vi "Begin Map.vi"   [LabVIEW 2017, in "LabPack.lvlib" / "Writer.lvclass"]
doc: "Starts writing and encoding a series of key-value pairs (ma) to MessagePack binary data format."
uses:
  Writer.lvclass
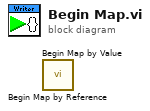
[diagram p0: block diagram]
diagram:
  n1 = call "Begin Map by Reference.vi"() -> ()  [unwired: 10 in, 2 out]
  n2 = call "Begin Map by Value.vi"() -> ()  [unwired: 10 in, 2 out]
